vi "LJM read open config.vi"(0 "Working Directory":path, 5 "filename":string="ljlogm_open.cfg") -> (4 "DeviceType":string="LJM_dtANY", 6 "ConnectionType":string="LJM_ctANY", 8 "Identifier":string="LJM_idANY", 15 "error out":errorcluster)   [LabVIEW 2021]
uses:
  <vilib>/Utility/config.llb/Read Key (String).vi
  <vilib>/Utility/config.llb/Write Key (String).vi
  <vilib>/Utility/config.llb/NI_LVConfig.lvlib
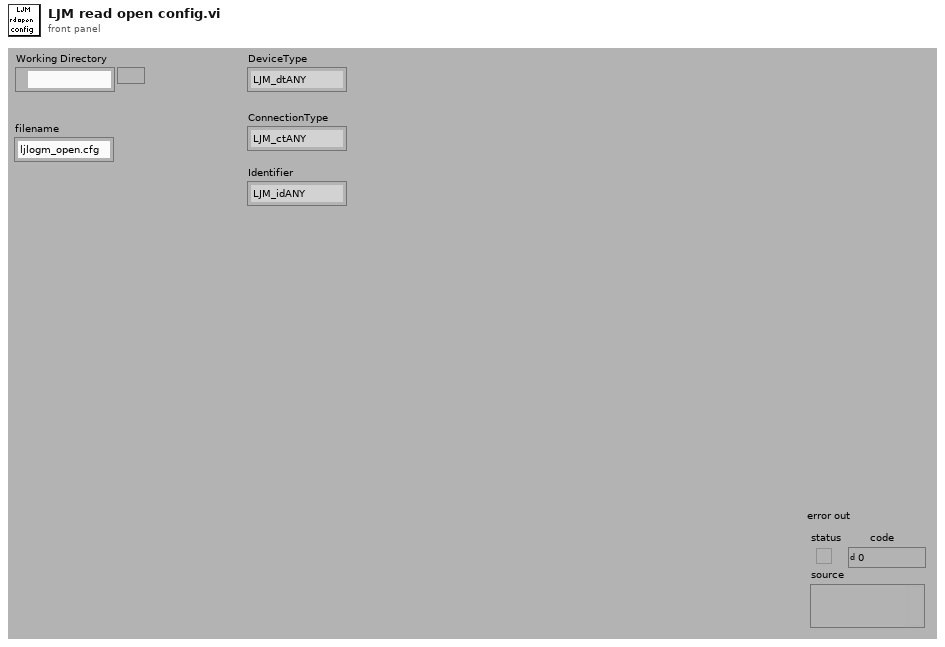
[diagram p1: front panel]
types:
  T1 = typedef "NI_LVConfig.lvlib/Config Data RefNum.ctl" = refnum<k1>
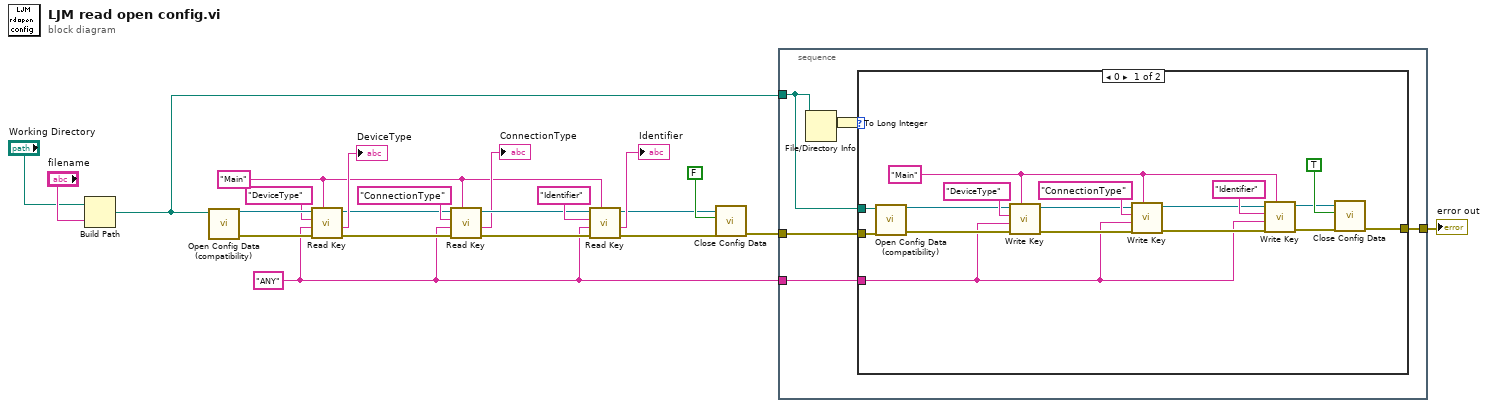
[diagram p0: block diagram]
diagram:
  w2 = "ANY" ("Data File Prefix")
  w5 = "Main" ("section")
  n1 = Build Path(base path="Working Directory", name or relative path="filename") -> (appended path=w3:path)
  n2 = call <vilib>:"Open Config Data (compatibility).vi"("configuration file path"=w3) -> ("error out"=w20:errorcluster, "refnum"=w21:T1)  [unwired: 8 in, 1 out]
  n3 = call-poly <vilib>:"Read Key.vi"("section"=w5, "error in (no error)"=w20, "default value"=w2, "key"="DeviceType", "refnum"=w21) -> ("error out"=w13:errorcluster, "value"=→"DeviceType":string, "refnum out"=w12:T1)  [unwired: 3 in, 1 out]
  n4 = call-poly <vilib>:"Read Key.vi"("section"=w5, "error in (no error)"=w13, "default value"=w2, "key"="ConnectionType", "refnum"=w12) -> ("error out"=w11:errorcluster, "value"=→"ConnectionType":string, "refnum out"=w10:T1)  [unwired: 3 in, 1 out]
  n5 = call-poly <vilib>:"Read Key.vi"("section"=w5, "error in (no error)"=w11, "default value"=w2, "key"="Identifier", "refnum"=w10) -> ("error out"=w6:errorcluster, "value"=→"Identifier":string, "refnum out"=w7:T1)  [unwired: 3 in, 1 out]
  n6 = call <vilib>:"Close Config Data.vi"("error in (no error)"=w6, "write file if changed (T)"=FALSE ("write configuration file? (F)"), "refnum"=w7) -> ("error out"=w4:errorcluster)  [unwired: 7 in, 1 out]
  n7 = stacked-sequence {
    tunnel: w4 -> [w27]
    tunnel: w3 -> [w26]
    tunnel: w2 -> [w25]
    tunnel: [w24] -> w1
    frame #0 {
      n8 = File/Directory Info(path=w26) -> (size=w23:i64)  [unwired: 1 in, 6 out]
      n9 = To Long Integer(number=w23) -> (32bit integer=w28:i32)
      n10 = case shown="0" w28 {
        tunnel: w27 -> [w44 w46]
        tunnel: w26 -> [w43 _]
        tunnel: w25 -> [w34 _]
        tunnel: [w32 w46] -> w24
        frame 0 {
          w33 = "Main" ("section")
          n11 = call <vilib>:"Open Config Data (compatibility).vi"("error in (no error)"=w44, "configuration file path"=w43) -> ("error out"=w41:errorcluster, "refnum"=w42:T1)  [unwired: 7 in, 1 out]
          n12 = call-poly <vilib>:"Write Key.vi"("section"=w33, "error in (no error)"=w41, "value"=w34, "key"="DeviceType", "refnum"=w42) -> ("error out"=w37:errorcluster, "refnum out"=w31:T1)  [unwired: 4 in, 1 out]
          n13 = call-poly <vilib>:"Write Key.vi"("section"=w33, "error in (no error)"=w37, "value"=w34, "key"="ConnectionType", "refnum"=w31) -> ("error out"=w36:errorcluster, "refnum out"=w30:T1)  [unwired: 4 in, 1 out]
          n14 = call-poly <vilib>:"Write Key.vi"("section"=w33, "error in (no error)"=w36, "value"=w34, "key"="Identifier", "refnum"=w30) -> ("error out"=w35:errorcluster, "refnum out"=w29:T1)  [unwired: 4 in, 1 out]
          n15 = call <vilib>:"Close Config Data.vi"("error in (no error)"=w35, "write file if changed (T)"=TRUE ("write configuration file? (F)"), "refnum"=w29) -> ("error out"=w32:errorcluster)  [unwired: 7 in, 1 out]
        }
        frame 1, Default {
        }
      }
    }
  }
  "error out" <- w1
